vi "Manhattan Distance.vi"(6 "y 2":i32, 9 "x 2":i32, 10 "x":i32, 11 "y":i32) -> (3 "Manhattan Distance":i32)   [LabVIEW 2019]
doc: "Compute Manhattan Distance between two point:\n\n|x1 - x2| + |y1 - y2|"
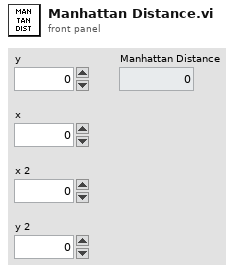
[diagram p1: front panel]
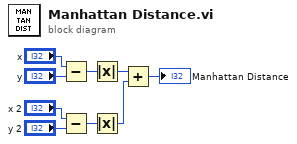
[diagram p0: block diagram]
diagram:
  n1 = Subtract(x="x", y="y") -> (x-y=w1:i32)
  n2 = Subtract(x="x 2", y="y 2") -> (x-y=w6:i32)
  n3 = Absolute Value(x=w1) -> (abs(x)=w7:i32)
  n4 = Absolute Value(x=w6) -> (abs(x)=w8:i32)
  n5 = Add(x=w7, y=w8) -> (x+y=→"Manhattan Distance":i32)
